vi "Start-Stop_edge2.vi"(11 "TriggerSn":bool) -> (0 "Stop_Tn [s]":dbl format="%#_20g", 1 "Start_Tn [s]":dbl format="%#_20g", 5 "TriggerSn_prev0":bool, 7 "TriggerSn_prev-1":bool)   [LabVIEW 2020]
doc: "Get Rise and Fall edge in [ms] of trigger signal input."
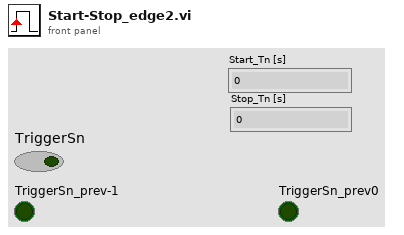
[diagram p1: front panel]
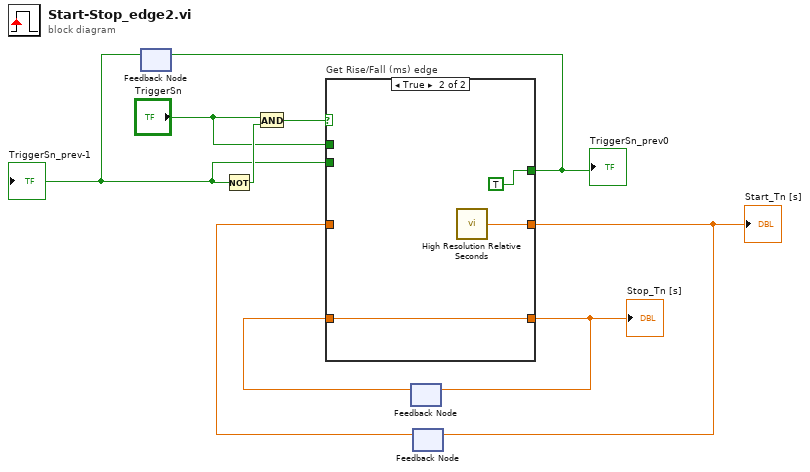
[diagram p0: block diagram]
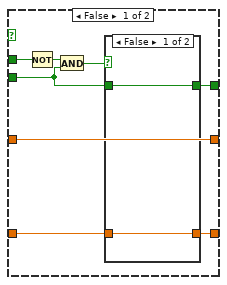
[diagram p2: hidden frame]
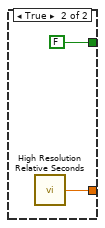
[diagram p3: hidden frame]
diagram:
  n1 = feedback #1() -> (w6:bool)  [unwired: 1 in]
  "TriggerSn_prev-1" <- w6
  n2 = Not(x=w6) -> (.not. x?=w9:bool)
  n3 = And(x="TriggerSn", y=w9) -> (x .and. y?=w8:bool)
  n4 = feedback #2() -> (w3:dbl)  [unwired: 1 in]
  n5 = feedback #3() -> (w1:dbl)  [unwired: 1 in]
  n6 = case "Get Rise/Fall (ms) edge" shown="True" w8 {
    tunnel: [w10 w24] -> w2
    tunnel: [w13 TRUE] -> w5
    tunnel: w1 -> [w10 _]
    tunnel: w3 -> [w11 w22]
    tunnel: [w14 w22] -> w4
    tunnel: "TriggerSn" -> [w17 _]
    tunnel: w6 -> [w12 _]
    frame False {
      n7 = Not(x=w17) -> (.not. x?=w16:bool)
      n8 = And(x=w16, y=w12) -> (x .and. y?=w15:bool)
      n9 = case shown="False" w15 {
        tunnel: [w18 w21] -> w14
        tunnel: [w19 FALSE] -> w13
        tunnel: w12 -> [w19 _]
        tunnel: w11 -> [w18 _]
        frame False {
        }
        frame True {
          n10 = call <vilib>:"High Resolution Relative Seconds.vi"() -> ("relative seconds"=w21:dbl)
        }
      }
    }
    frame True {
      n11 = call <vilib>:"High Resolution Relative Seconds.vi"() -> ("relative seconds"=w24:dbl)
    }
  }
  "TriggerSn_prev0" <- w5
  "Start_Tn [s]" <- w2
  "Stop_Tn [s]" <- w4
  n12 = feedback-in #1(w5) -> ()
  n13 = feedback-in #2(w4) -> ()
  n14 = feedback-in #3(w2) -> ()
